vi "ErrorWrite.vi"(6 "Error to write":errorcluster, 8 "error in":errorcluster, 9 "time":timestamp, 10 "string":string, 11 "TerminalIn":T1) -> (0 "error out":errorcluster, 3 "TerminalOut":T1)   [LabVIEW 2021, in "LibDan.lvlib"]
uses:
  LibDan.lvlib
  TerminalDef.ctl
  <vilib>/Utility/config.llb/Config Data RefNum.ctl
  <vilib>/Utility/error.llb/DialogType.ctl
  <vilib>/MultiError/TokenizeJSON/Multi Error Cluster.lvlib
  <vilib>/Utility/config.llb/NI_LVConfig.lvlib
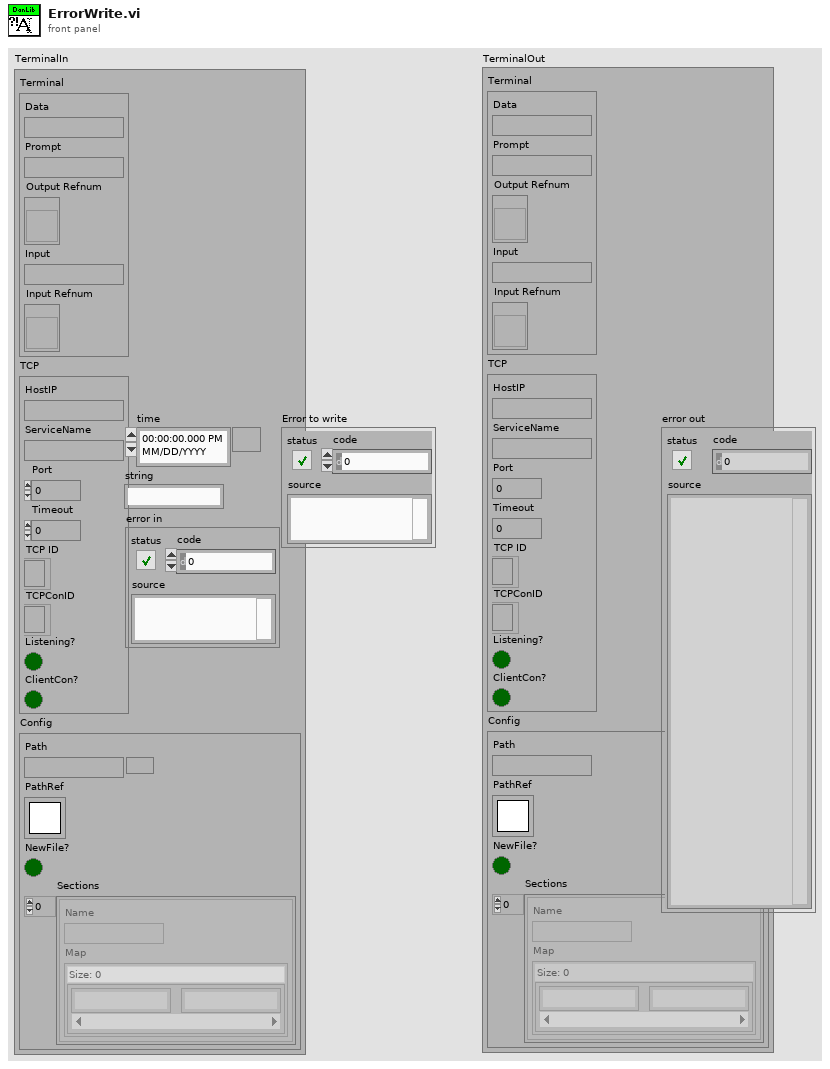
[diagram p1: front panel]
types:
  T1 = typedef "LibDan.lvlib/TerminalDef.ctl" = cluster{"Terminal":cluster{"Data":string, "Prompt":string, "Output Refnum":refnum<vi>, "Input":string, "Input Refnum":refnum<vi>}, "TCP":cluster{"HostIP":string, "ServiceName":string, "Port":u16, "Timeout":i32, "TCP ID":refnum<k5>, "TCPConID":refnum<k5>, "Listening?":bool, "ClientCon?":bool}, "Config":cluster{"Path":path, "PathRef":T2, "NewFile?":bool, "Sections":cluster{"Name":string, "Map":map{string, string}}[]}}
  T2 = typedef "NI_LVConfig.lvlib/Config Data RefNum.ctl" = refnum<k1>
  T3 = typedef "DialogType.ctl" = u16
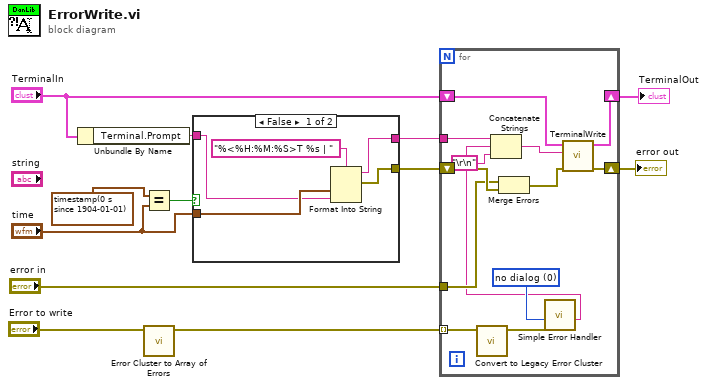
[diagram p0: block diagram]
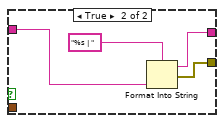
[diagram p2: hidden frame]
diagram:
  n1 = Unbundle By Name("TerminalIn") -> ("Terminal.Prompt"=w6:string)
  n2 = Equal?(x=timestamp(0 s since 1904-01-01), y="time") -> (x = y?=w10:bool)
  n3 = call <vilib>:"Error Cluster to Array of Errors.vi"("error"="Error to write") -> ("array of errors"=w1:errorcluster[])  [unwired: 10 in]
  n4 = case shown="False" w10 {
    tunnel: [w17 w21] -> w4
    tunnel: "time" -> [w15 _]
    tunnel: w6 -> [w14 w19]
    tunnel: [w13 w18] -> w5
    frame False {
      n5 = Format Into String(format string="%<%H:%M:%S>T %s | ", w15, w14) -> (resulting string=w13:string, error out=w17:errorcluster)  [unwired: 2 in]
    }
    frame True {
      n6 = Format Into String(format string="%s | ", w19) -> (resulting string=w18:string, error out=w21:errorcluster)  [unwired: 2 in]
    }
  }
  n7 = for {
    tunnel: w5 -> [w30]
    tunnel: "error in" -> [w27]
    shift-right: [w34] -> w12
    shift-left: "TerminalIn" -> [w32]
    shift-right: [w33] -> w11
    shift-left: w4 -> [w28]
    tunnel: w1 -> [w24] mode=indexing
    w25 = T3 0 items=["no dialog", "OK message", "continue or stop message", "OK message + warnings", "continue/stop + warnings"] ("type of dialog (OK msg:1)")
    n8 = call <vilib>:"Convert to Legacy Error Cluster.vi"("error in"=w24) -> ("error out"=w23:errorcluster)  [unwired: 10 in]
    n9 = Merge Errors(w27, w28) -> (w29:errorcluster)
    n10 = call <vilib>:"Simple Error Handler.vi"("type of dialog (OK msg:1)"=w25, "error in (no error)"=w23) -> ("source out"=w22:string)  [unwired: 3 in, 4 out]
    n11 = Concatenate Strings(w30, w22, "\r\n") -> (w31:string)
    n12 = call "TerminalWrite.vi"("error in"=w29, "string"=w31, "TerminalIn"=w32) -> ("error out"=w33:errorcluster, "TerminalOut"=w34:T1)  [unwired: 7 in]
  }
  "TerminalOut" <- w12
  "error out" <- w11
